vi "Register Value.vi"(1 "Register":T1 items=["PV"=0, "SV"=5, "P1"=24, "I1"=25, "D1"=26]) -> (0 "RegAddr (Hex)":u16 format="%x")   [LabVIEW 2023, in "PIDModbus.lvlib"]
uses:
  PIDModbus.lvlib
  Controls/Register Enum.ctl
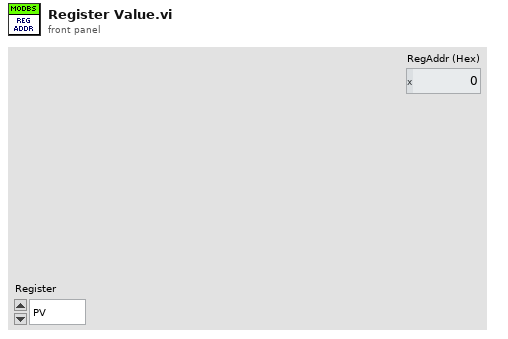
[diagram p1: front panel]
types:
  T1 = typedef "PIDModbus.lvlib/Register Enum.ctl" = u16
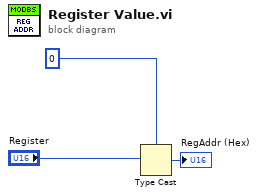
[diagram p0: block diagram]
diagram:
  n1 = Type Cast(type=u16 0, x="Register") -> (*(type *) &x=→"RegAddr (Hex)":u16)
